vi "TDMSDataSaver.vi"(4 "error In":errorcluster, 5 "Good to drive? Data":waveform(dbl)[](array[waveform]), 6 "Alcohol Levels Data":waveform(dbl)[](array[waveform]), 7 "Who is doing the test?":string) -> (0 "error out":errorcluster)   [LabVIEW 2019]
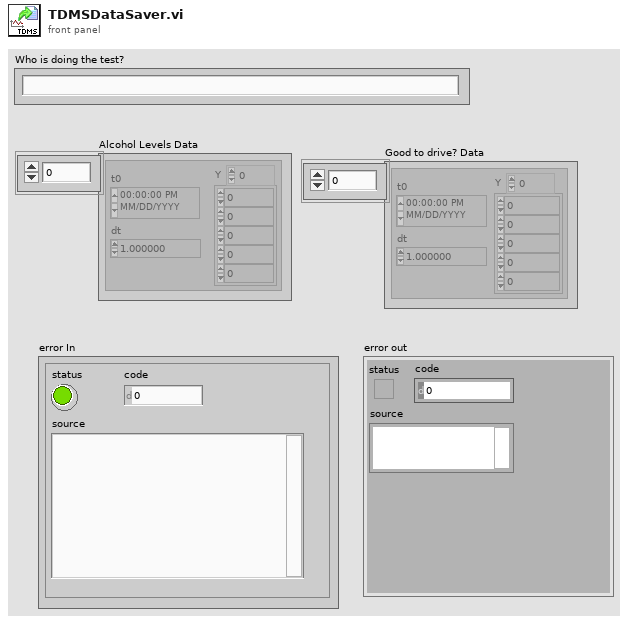
[diagram p1: front panel]
types:
  T1 = enum16{"open", "open or create", "create or replace", "create", "open (read-only)"}
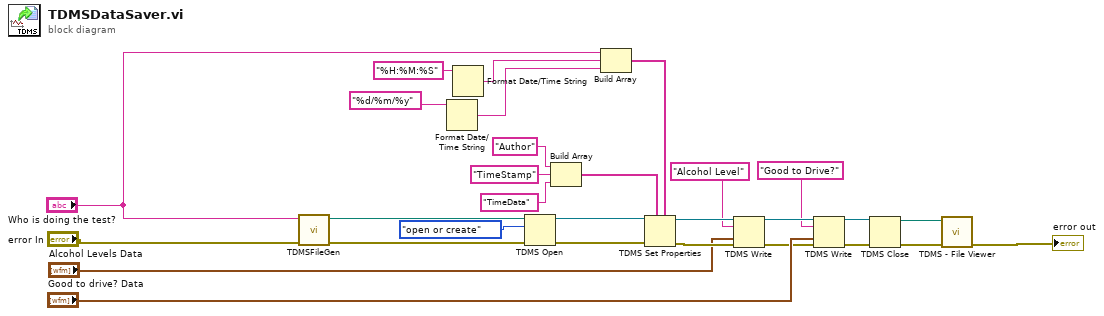
[diagram p0: block diagram]
diagram:
  n1 = call "TDMSFileGen.vi"("error in (no error)"="error In", "Who is doing the test?"="Who is doing the test?") -> ("error out"=w27:errorcluster, "appended path"=w26:path)  [unwired: 8 in]
  n2 = Format Date/Time String(time format string (%c)="%d/%m/%y") -> (date/time string=w15:string)  [unwired: 2 in]
  n3 = Format Date/Time String(time format string (%c)="%H:%M:%S") -> (date/time string=w17:string)  [unwired: 2 in]
  n4 = TDMS Open(8:w27, 10:T1."open or create" ("operation (0:open)"), 11:w26) -> (0:w25:errorcluster, 3:w24:refnum<k34>)  [unwired: 4 in]
  n5 = Build Array("Author" ("initial string"), "TimeStamp" ("initial string"), "TimeData" ("initial string")) -> (w20:string[])
  n6 = Build Array("Who is doing the test?", w17, w15) -> (w14:string[])
  n7 = TDMS Set Properties(5:w14, 7:w20, 8:w25, 11:w24) -> (0:w11:errorcluster, 3:w13:refnum<k34>)  [unwired: 2 in, 2 out]
  n8 = TDMS Write(0:w13, 5:"Alcohol Level" ("group name in (Untitled)"), 9:"Alcohol Levels Data", 11:w11) -> (4:w9:refnum<k34>, 15:w2:errorcluster)  [unwired: 2 in, 2 out]
  n9 = TDMS Write(0:w9, 5:"Good to Drive?" ("group name in (Untitled)"), 9:"Good to drive? Data", 11:w2) -> (4:w6:refnum<k34>, 15:w1:errorcluster)  [unwired: 2 in, 2 out]
  n10 = TDMS Close(8:w1, 11:w6) -> (0:w7:errorcluster, 3:w8:path)
  n11 = call <vilib>:"TDMS - File Viewer.vi"("error in (no error)"=w7, "file path"=w8) -> ("error out"=→"error out":errorcluster)  [unwired: 4 in, 1 out]
